vi "DesiredLevelWrite.vi"   [LabVIEW 2014]
uses:
  ElevatorStates.ctl
  Global Data!!!.vi
types:
  T1 = typedef "ElevatorStates.ctl" = enum16{"DropSequence", "Reset", "Drop1Stage", "2StageEngage", "Lift1Stage", "1StageEngage", "Rest", "InterruptedLift", "Manual", "Auto2Man"}
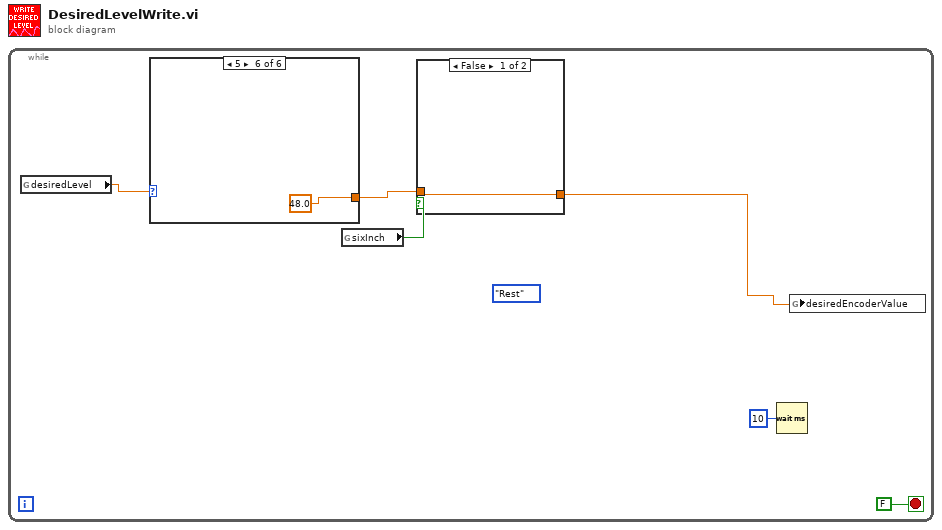
[diagram p0: block diagram]
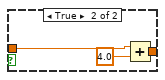
[diagram p2: hidden frame]
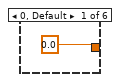
[diagram p3: hidden frame]
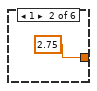
[diagram p4: hidden frame]
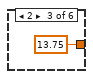
[diagram p5: hidden frame]
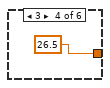
[diagram p6: hidden frame]
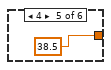
[diagram p7: hidden frame]
diagram:
  n1 = while {
    stop <- FALSE stop-if-true
    (unwired) ElevatorStates."Rest" ("Enum")
    n2 = global read "Global Data!!!.vi" "desiredLevel"() -> (w6:dbl)
    n3 = case shown="5" w6 {
      tunnel: [0.0 2.75 13.75 26.5 38.5 48.0] -> w4
      frame 0, Default {
      }
      frame 1 {
      }
      frame 2 {
      }
      frame 3 {
      }
      frame 4 {
      }
      frame 5 {
      }
    }
    n4 = global read "Global Data!!!.vi" "sixInch"() -> (w5:bool)
    n5 = case shown="False" w5 {
      tunnel: w4 -> [w7 w10]
      tunnel: [w7 w8] -> w1
      frame False {
      }
      frame True {
        n6 = Add(x=w10, y=4.0) -> (x+y=w8:dbl)
      }
    }
    n7 = Wait (ms)(milliseconds to wait=u32 10) -> ()  [unwired: 1 out]
    n8 = global write "Global Data!!!.vi" "desiredEncoderValue"(w1) -> ()
  }
